vi "Read Xbox Triggers.vi"(8 "error in (no error)":errorcluster, 11 "XBoxController in":refnum<class "XBoxController.lvclass">) -> (0 "error out":errorcluster, 2 "Xbox Triggers":T2 {"Right Trigger" scale=0.0..1.0; "Left Trigger" scale=0.0..1.0}, 3 "XBoxController out":refnum<class "XBoxController.lvclass">)   [LabVIEW 2013, in "XBoxController.lvclass"]
uses:
  XBoxController.lvclass
  XBoxController.lvclass/XBoxController.ctl
panel:
  in  "Trigger Threshold":dbl(knob)=0.8999999999999999 step=0.1 scale=0.1..0.9
  out "Axes":T1
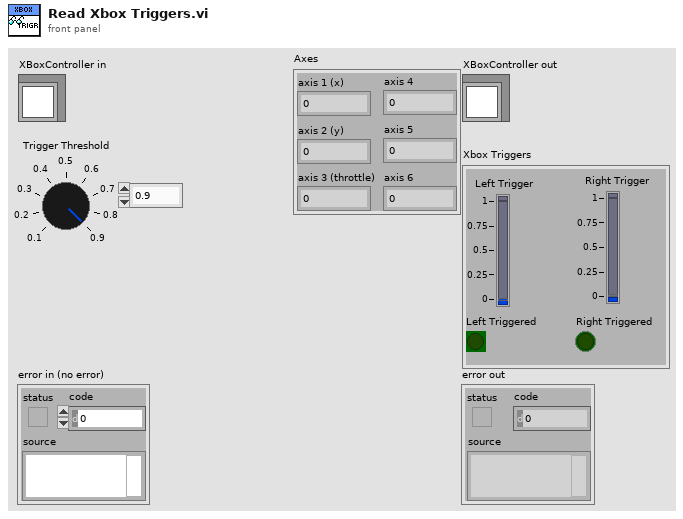
[diagram p1: front panel]
types:
  T1 = cluster{"axis 1 (x)":dbl, "axis 2 (y)":dbl, "axis 3 (throttle)":dbl, "axis 4":dbl, "axis 5":dbl, "axis 6":dbl}
  T2 = cluster{"Left Trigger":dbl, "Right Trigger":dbl, "Left Triggered":bool, "Right Triggered":bool}
  T3 = typedef "WPI_JoystickDevRef.ctl" = cluster{"Device":T4}
  T4 = typedef "WPI_JoystickDeviceEnum.ctl" = enum16{"USB 1", "USB 2", "USB 3", "USB 4", "Kinect 1", "Kinect 2"}
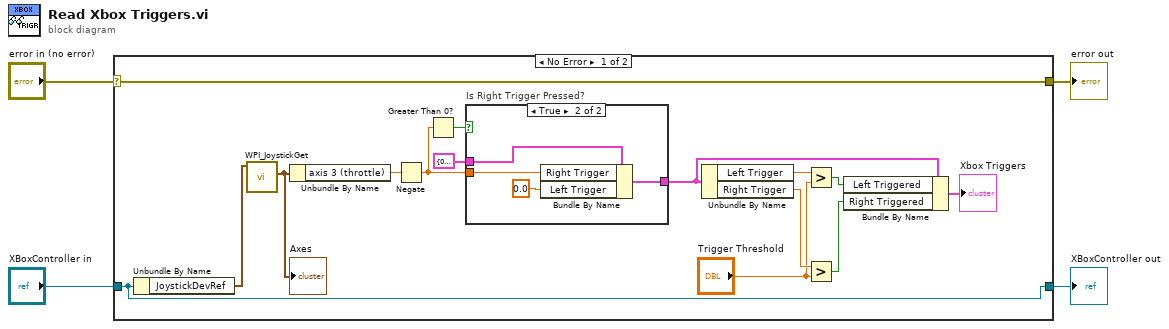
[diagram p0: block diagram]
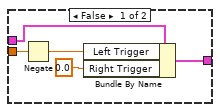
[diagram p2: hidden frame]
diagram:
  n1 = case shown="No Error" "error in (no error)" {
    selector: "error in (no error)" -> [w19 w29]
    tunnel: [w19 w29] -> w3
    tunnel: [w18 w30] -> w1
    tunnel: "XBoxController in" -> [w18 w30]
    frame No Error {
      n2 = Unbundle By Name(w18) -> ("JoystickDevRef"=w17:T3)
      n3 = call <vilib>:"WPI_JoystickGet.vi"("JoystickDevRef"=w17) -> ("Axes"=w16:T1)  [unwired: 4 in, 2 out]
      "Axes" <- w16
      n4 = Unbundle By Name(w16) -> ("axis 3 (throttle)"=w14:dbl)
      n5 = Negate(x=w14) -> (-x=w6:dbl)
      n6 = Greater Than 0?(x=w6) -> (x > 0?=w15:bool)
      n7 = case "Is Right Trigger Pressed?" shown="True" w15 {
        tunnel: w6 -> [w23 w28]
        tunnel: [w20 w27] -> w12
        tunnel: T2 {"Left Trigger"=0.0, "Right Trigger"=0.0, "Left Triggered"=FALSE, "Right Triggered"=FALSE} ("Xbox Triggers") -> [w24 w26]
        frame False {
          n8 = Negate(x=w23) -> (-x=w22:dbl)
          n9 = Bundle By Name(cluster=w24, "Left Trigger"=w22, "Right Trigger"=0.0) -> (w20:T2)
        }
        frame True {
          n10 = Bundle By Name(cluster=w26, "Right Trigger"=w28, "Left Trigger"=0.0) -> (w27:T2)
        }
      }
      n11 = Unbundle By Name(w12) -> ("Left Trigger"=w11:dbl, "Right Trigger"=w9:dbl)
      n12 = Greater?(x=w11, y="Trigger Threshold") -> (0:w10:bool)
      n13 = Greater?(x=w9, y="Trigger Threshold") -> (0:w7:bool)
      n14 = Bundle By Name(cluster=w12, "Left Triggered"=w10, "Right Triggered"=w7) -> (→"Xbox Triggers":T2)
    }
    frame Error {
    }
  }
  "error out" <- w3
  "XBoxController out" <- w1
